vi "Mean and SD.vi"(11 "JSON Object In":refnum<class "JSON Object.lvclass">) -> (1 "SD":refnum<class "JSON Scalar.lvclass">, 2 "Is SD":bool, 3 "JSON Value":refnum<class "JSON Value.lvclass">)   [LabVIEW 2020, in "Library Commun.lvlib" / "JSON Object.lvclass"]
uses:
  JSON Object.lvclass
  C:/Users/ngarcin/OneDrive - Altyor/Standard TB/Class/JSON API/JSON Value/JSON Value.lvclass
  JSON Value/JSON Value.lvclass
  JSON Scalar/JSON Scalar.lvclass
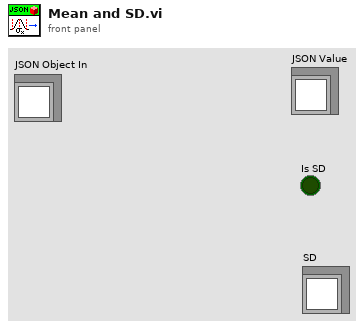
[diagram p1: front panel]
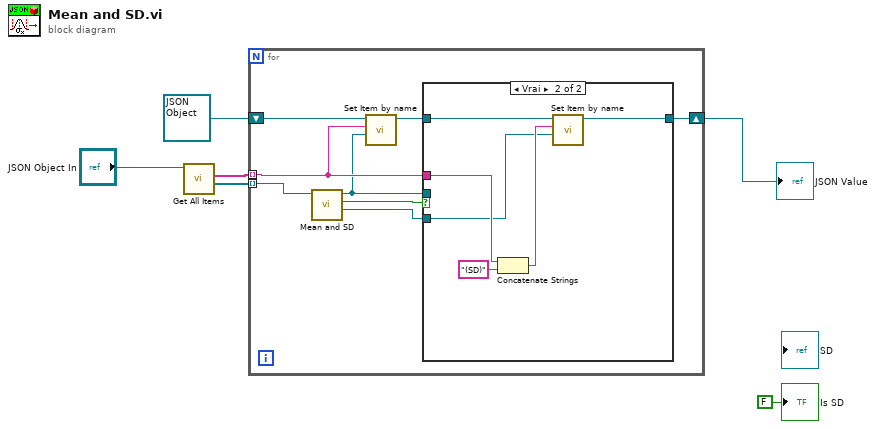
[diagram p0: block diagram]
diagram:
  n1 = call-dynamic "Get All Items.vi"("JSON Object in"="JSON Object In") -> ("Values"=w4:refnum<class "JSON Value.lvclass">[], "Item Names"=w3:string[])  [unwired: 7 in, 2 out]
  n2 = for {
    tunnel: w4 -> [w14] mode=indexing
    tunnel: w3 -> [w9] mode=indexing
    shift-right: [w7] -> w1
    shift-left: refnum<class "JSON Object.lvclass"> refnum ("JSON Object In") -> [w10]
    n3 = call-dynamic "Mean and SD.vi"("Statistics in"=w14) -> ("SD"=w12:refnum<class "JSON Scalar.lvclass">, "Is SD"=w13:bool, "Mean and Standard Deviation(SD)"=w8:refnum<class "JSON Value.lvclass">)  [unwired: 8 in]
    n4 = call-dynamic "Set Item by name.vi"("Value"=w8, "name"=w9, "JSON Object in"=w10) -> ("JSON Object out"=w11:refnum<class "JSON Object.lvclass">)  [unwired: 6 in, 2 out]
    n5 = case shown="Vrai" w13 {
      tunnel: w12 -> [_ w17]
      tunnel: w9 -> [_ w19]
      tunnel: w8 -> [_ _]
      tunnel: w11 -> [w15 w20]
      tunnel: [w15 w16] -> w7
      frame False {
      }
      frame True {
        n6 = Concatenate Strings(w19, "(SD)" ("string")) -> (w18:string)
        n7 = call-dynamic "Set Item by name.vi"("Value"=w17, "name"=w18, "JSON Object in"=w20) -> ("JSON Object out"=w16:refnum<class "JSON Object.lvclass">)  [unwired: 6 in, 2 out]
      }
    }
  }
  "JSON Value" <- w1
  "Is SD" <- FALSE ("Is SD")
